vi "DialogInput.vi"(11 "string initialization":string) -> (2 "True?":bool, 3 "email":string)   [LabVIEW 2010]
panel:
  in  "Enter an email address":string
  in  "Cancel":bool
  in  "Ok":bool
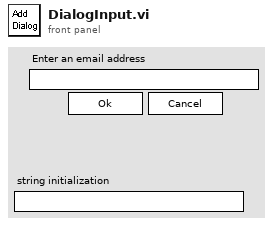
[diagram p1: front panel]
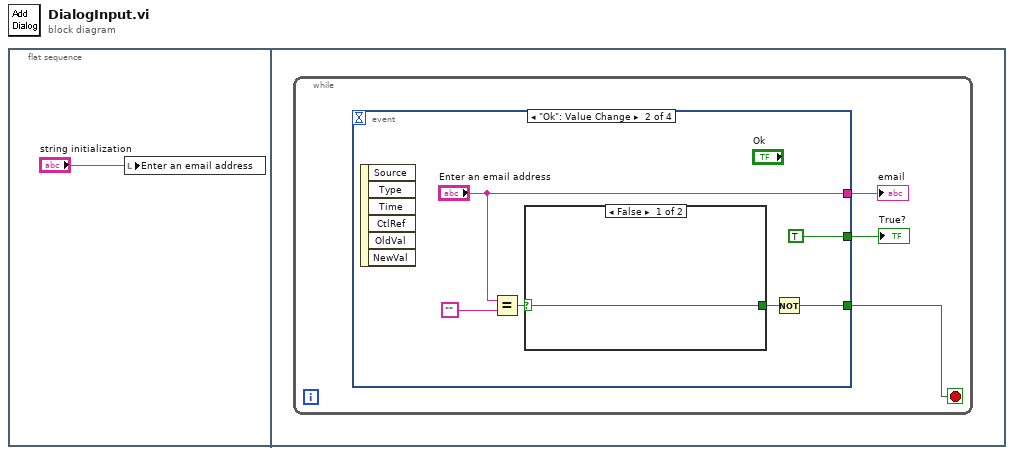
[diagram p0: block diagram]
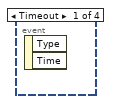
[diagram p2: hidden frame]
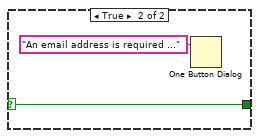
[diagram p3: hidden frame]
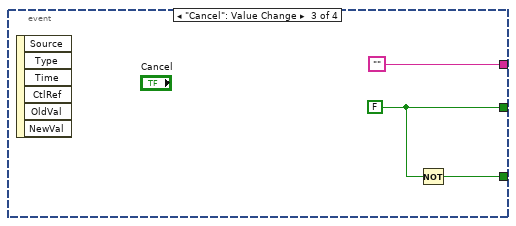
[diagram p4: hidden frame]
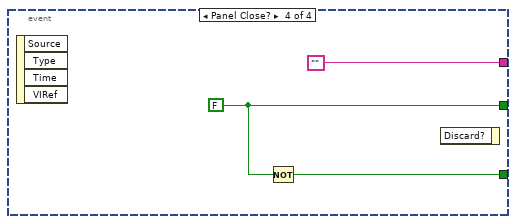
[diagram p5: hidden frame]
diagram:
  n1 = flat-sequence {
    frame #0 {
      n2 = local write "Enter an email address"("string initialization") -> ()
    }
    frame #1 {
      n3 = while {
        stop <- w2 stop-if-true
        n4 = event shown="[1] \"Ok\": Value Change" {
          selector: _ -> [_ _ _ _]
          dyn-events: _ -> [_ _ _ _]
          timeout: _ -> [_ _ _ _]
          tunnel: [_ "Enter an email address" "" ""] -> w4
          tunnel: [_ TRUE ("Ok") w14 w18] -> w3
          tunnel: [_ w5 w15 w17] -> w2
          event Timeout {
            n5 = event-data() -> ()  [unwired: 3 out]
          }
          event "Ok": Value Change {
            n6 = event-data() -> ()  [unwired: 7 out]
            n7 = Equal?(x="Enter an email address", y="") -> (x = y?=w7:bool)
            n8 = case shown="False" w7 {
              selector: w7 -> [w11 w12]
              tunnel: [w11 w12] -> w6
              frame False {
              }
              frame True {
                n9 = One Button Dialog(message="An email address is required ...") -> ()  [unwired: 2 out]
              }
            }
            n10 = Not(x=w6) -> (.not. x?=w5:bool)
          }
          event "Cancel": Value Change {
            w14 = FALSE ("Ok")
            n11 = event-data() -> ()  [unwired: 7 out]
            n12 = Not(x=w14) -> (.not. x?=w15:bool)
          }
          event Panel Close? {
            w18 = FALSE ("Ok")
            n13 = event-data() -> ()  [unwired: 5 out]
            n14 = Not(x=w18) -> (.not. x?=w17:bool)
            n15 = event-data() -> ()  [unwired: 1 in, 2 out]
          }
        }
        "email" <- w4
        "True?" <- w3
      }
    }
  }
